vi "Write Image File (ARGB).vi"(8 "error in (no error)":errorcluster, 10 "Filepath in":path, 11 "ARGB Image Source in":T1) -> (0 "error out":errorcluster, 3 "Filepath":path)   [LabVIEW 2020, in "image.lvlib"]
doc: "Write an Image file. A broad range of file formats are supported including jpeg, bitmap, png, webp, tiff and others."
uses:
  image.lvlib
  ARGB Image.ctl
  9723f547-2605-4a38-b7b5-a8bc0a93fff0.vi
  <vilib>/Utility/error.llb/Error Cluster From Error Code.vi
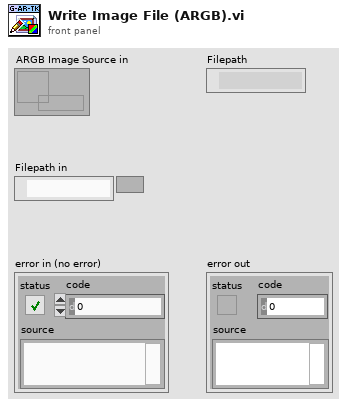
[diagram p1: front panel]
types:
  T1 = typedef "image.lvlib/ARGB Image.ctl" = refnum<data-value>
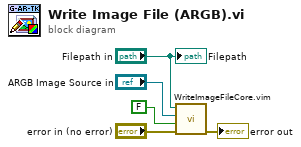
[diagram p0: block diagram]
diagram:
  n1 = call "WriteImageFileCore.vim"("error in (no error)"="error in (no error)", "SaveAlpha"=FALSE, "Src"="ARGB Image Source in", "Filepath"="Filepath in") -> ("error out"=→"error out":errorcluster)  [unwired: 7 in]
  "Filepath" <- "Filepath in"
